vi "EmailAttachment.vi"(8 "error in (no error)":errorcluster, 10 "Attachment path":string, 11 "Subject":string) -> ()   [LabVIEW 2022 SP3]
uses:
  <vilib>/Platform/browser.llb/Open URL in Default Browser (string).vi
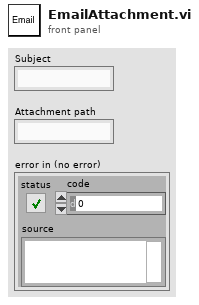
[diagram p1: front panel]
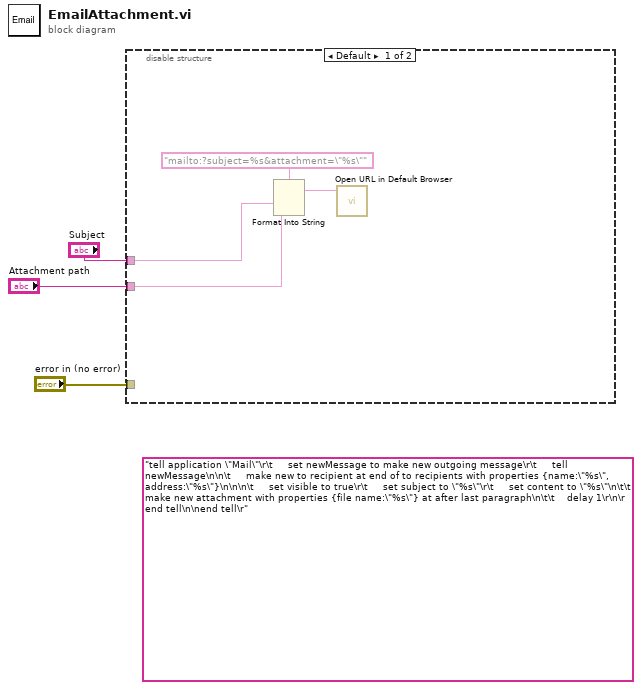
[diagram p0: block diagram]
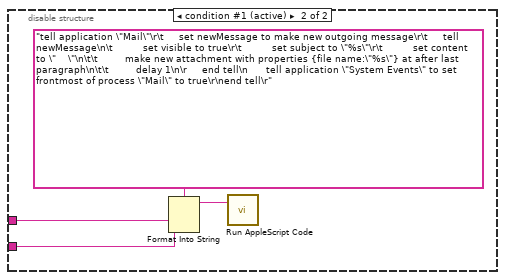
[diagram p2: hidden frame]
diagram:
  (unwired) "tell application \"Mail\"\r\t     set newMessage to make new outgoing message\r\t     tell newMessage\n\n\t     make new to recipient at end of to recipients with properties {name:\"%s\", address:\"%s\"}\n\n\n\t     set visible to true\r\t     set subject to \"%s\"\r\t     set content to \"%s\"\n\t\t    make new attachment with properties {file name:\"%s\"} at after last paragraph\n\t\t    delay 1\r\n\r     end tell\n\nend tell\r" ("input string")
  n1 = disable-structure shown="Default" {
    disable-tunnel: "Attachment path" -> [w6 w11]
    disable-tunnel: "error in (no error)" -> [_ _]
    disable-tunnel: "Subject" -> [w4 w8]
    frame condition #0 {
      n2 = Format Into String(format string="mailto:?subject=%s&attachment=\"%s\"", w4, w6) -> (resulting string=w5:string)  [unwired: 2 in, 1 out]
      n3 = call-poly <vilib>:"Open URL in Default Browser.vi"("URL"=w5) -> ()  [unwired: 5 in, 2 out]
    }
    frame condition #1 (active) {
      n4 = Format Into String(format string="tell application \"Mail\"\r\t     set newMessage to make new outgoing message\r\t     tell newMessage\n\t          set visible to true\r\t          set subject to \"%s\"\r\t          set content to \"    \"\n\t\t         make new attachment with properties {file name:\"%s\"} at after last paragraph\n\t\t         delay 1\n\r     end tell\n      tell application \"System Events\" to set frontmost of process \"Mail\" to true\r\nend tell\r" ("input string"), w8, w11) -> (resulting string=w10:string)  [unwired: 2 in, 1 out]
      n5 = call <vilib>:"Run AppleScript Code.vi"("input string"=w10) -> ()  [unwired: 8 in, 3 out]
    }
  }
